vi "XY Graph Get Plots Metadata.vi"(8 "Error In":errorcluster, 11 "XYGraph Refnum":T1) -> (0 "Error Out":errorcluster, 1 "Plots Metadata Found?":bool, 2 "Plots Metadata":variant[](array[variant]), 3 "XYGraph Refnum":T1)   [LabVIEW 2019, in "XY Graph Add-Ons.lvlib"]
uses:
  XY Graph Add-Ons.lvlib
  XY Graph Refnum.ctl
  XY Graph Property Tag List.ctl
  <vilib>/UserTags/UserTags.lvlib
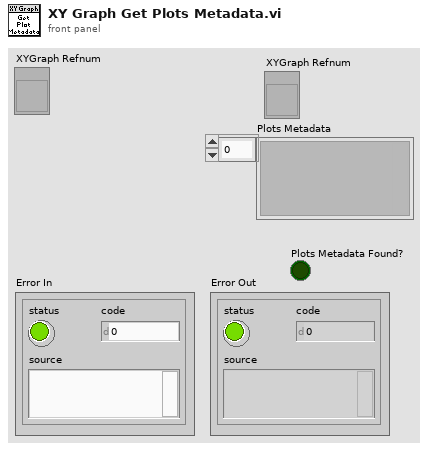
[diagram p1: front panel]
types:
  T1 = typedef "XY Graph Add-Ons.lvlib/XY Graph Refnum.ctl" = refnum<vi>
  T2 = typedef "XY Graph Add-Ons.lvlib/XY Graph Property Tag List.ctl" = enum16{"Max Legend Size", "Preserved Plots", "XScales.GridColors", "YScales.GridColors", "TipStrip String", "TipStrip Visible", "Tool Panels Visibility", "Plots Metadata"}
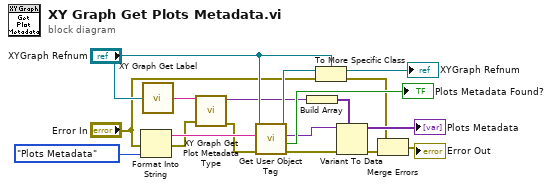
[diagram p0: block diagram]
diagram:
  n1 = Format Into String(error in="Error In", XY_Graph_Property_Tag_List."Plots Metadata" ("XY Graph Property Tag")) -> (resulting string=w14:string, error out=w6:errorcluster)  [unwired: 2 in]
  n2 = call "XY Graph Get Label.vi"("XYGraph"="XYGraph Refnum") -> ("Graph Label"=w8:string)  [unwired: 8 in]
  n3 = call "XY Graph Get Plot Metadata Type.vi"("Error In"=w6, "Graph Label"=w8) -> ("Error Out"=w5:errorcluster, "Plot Metadata Type"=w7:variant)  [unwired: 7 in, 1 out]
  n4 = call <vilib>:"Get User Object Tag.vi"("error in (no error)"=w5, "Tag Name"=w14, "Generic Refnum"="XYGraph Refnum") -> ("error out"=w12:errorcluster, "Was Tag Found?"=→"Plots Metadata Found?":bool, "Value"=w13:variant, "dup Generic Refnum"=w17:refnum<vi>)  [unwired: 5 in]
  n5 = Build Array(w7) -> (w4:variant[])
  n6 = To More Specific Class(target class="XYGraph Refnum", reference=w17, error in="Error In") -> (specific class reference=→"XYGraph Refnum":T1, error out=w2:errorcluster)
  n7 = Variant To Data(error in=w12, type=w4, Variant=w13) -> (data=→"Plots Metadata":variant[], error out=w10:errorcluster)
  n8 = Merge Errors(w2, w10) -> (→"Error Out":errorcluster)
